vi "Is Unset.vi"(4 "Config Element in":refnum<class "Config Element.lvclass">) -> (7 "Unset":bool)   [LabVIEW 2023, in "CDM-Config.lvlib" / "Config Element.lvclass"]
uses:
  Config Element.lvclass
  Config Element.lvclass/Config Element.ctl
  Node Info.ctl
  CDM-Config.lvlib
  Meta Data.ctl
  Value Type.ctl
  Element Data.ctl
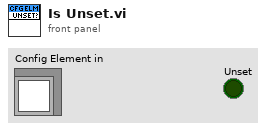
[diagram p1: front panel]
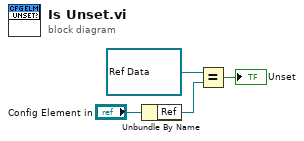
[diagram p0: block diagram]
diagram:
  n1 = Unbundle By Name("Config Element in") -> ("Ref"=w3:refnum<data-value>)
  n2 = Equal?(x=refnum<data-value> refnum, y=w3) -> (x = y?=→"Unset":bool)
